vi "Read Error Count.vi"(11 "Method Result In":T1) -> (2 "Error count":i32, 3 "Method Result Out":T1)   [LabVIEW 2020, in "Method Result.lvlib"]
uses:
  Method Result.lvlib
  Assertion Result/Public/TypeDefs/Status.ctl
  Assertion Result/Assertion Result.lvlib
  Assertion Result/Public/TypeDefs/Assertion Type.ctl
  Core/Result/Result.lvlib
  Assertion Result/Assertion Result.ctl
  Method Result.ctl
  Core/Result/Status.ctl
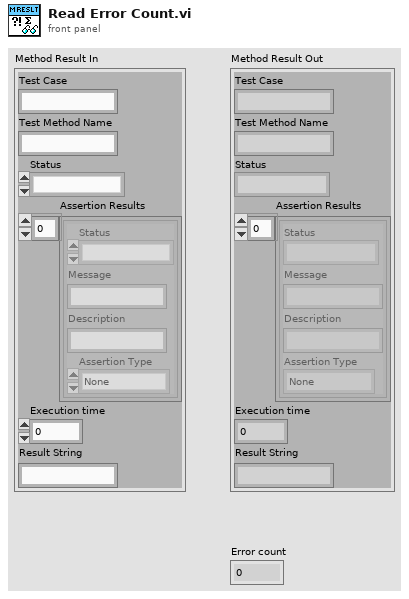
[diagram p1: front panel]
types:
  T1 = typedef "Method Result.lvlib/Method Result.ctl" = cluster{"Test Case":string, "Test Method Name":string, "Status":T2, "Assertion Results":T3[], "Execution time":dbl, "Result String":string}
  T2 = typedef "Result.lvlib/Status.ctl" = enum16{"", "Passed", "Failed", "Error", "Skipped", "Setup Error", "Broken", "Teardown Error"}
  T3 = typedef "Assertion Result.lvlib/Assertion Result.ctl" = cluster{"Status":T2, "Message":string, "Description":string, "Assertion Type":T4}
  T4 = typedef "Result.lvlib/Assertion Type.ctl" = enum16{"None", "Pass", "Fail", "Skip", "Pass if Equal", "Fail if Equal", "Pass if Error", "Fail if Error", "Pass if", "Fail if"}
  T5 = typedef "Assertion Result.lvlib/Status.ctl" = enum16{"Pass", "Fail", "Error", "Skipped", "Setup Error", "Broken", "Teardown Error"}
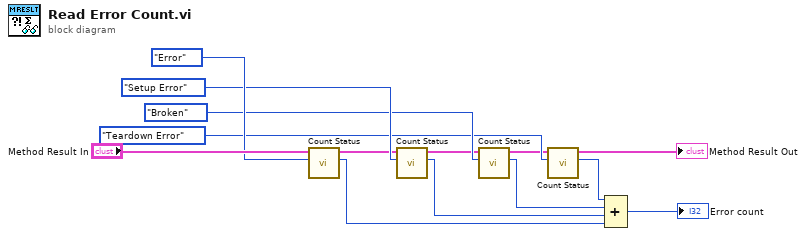
[diagram p0: block diagram]
diagram:
  n1 = call "Count Status.vi"("Status"=Status."Error", "Method Result in"="Method Result In") -> ("Count"=w3:i32, "Method Result out"=w9:T1)  [unwired: 8 in]
  n2 = call "Count Status.vi"("Status"=Status."Setup Error", "Method Result in"=w9) -> ("Count"=w4:i32, "Method Result out"=w8:T1)  [unwired: 8 in]
  n3 = call "Count Status.vi"("Status"=Status."Broken", "Method Result in"=w8) -> ("Count"=w5:i32, "Method Result out"=w7:T1)  [unwired: 8 in]
  n4 = call "Count Status.vi"("Status"=Status."Teardown Error", "Method Result in"=w7) -> ("Count"=w6:i32, "Method Result out"=→"Method Result Out":T1)  [unwired: 8 in]
  n5 = Compound Arithmetic op=ADD(w6, w5, w4, w3) -> (→"Error count":i32)
